vi "test.vi"() -> ()   [LabVIEW 2016]
uses:
  common_labview_tcpdevice/ts_labview_tcp/tcpTypedefs/TCPSettings.ctl
  IDome/domeTypedefs/azimuth.ctl
  domeCommunicator/ComTypedefs/shortStatus.ctl
  domeCommunicator/ComTypedefs/openingStates.ctl
  IDome/domeTypedefs/openingPercentage.ctl
  domeCommunicator/ComTypedefs/sensorCode.ctl
  domeCommunicator/ComTypedefs/azimimuthPositionStatus.ctl
  IDome/domeTypedefs/direction.ctl
  IDome/domeTypedefs/domeState.ctl
  IDome/domeTypedefs/motionDirection.ctl
  IDome/domeTypedefs/openingMotion.ctl
  domeCommunicator/ComTypedefs/engineeringStatus.ctl
  domeCommunicator/ATDomeCommunicator.lvclass
  domeController/DomeController.lvclass
  domeCommunicator/ComTypedefs/queries.ctl
  domeCommunicator/ComTypedefs/commands.ctl
panel:
  out "Timeout":errorcluster
  in  "TCP Settings":T1={"IP"="192.168.222.77", "port_low"=17310, "port_up"=17310, "connection_timeout "=1500, "reading_timeout"=1500, "writing_timeout"=1500}
  out "Connected":bool
  in  "disconnect":bool
  in  "connect":bool
  in  "azimuth":T2 min=0.0 max=360.0
  in  "SynchronizedClose":bool
  in  "MoveToAzimuth":bool
  in  "Synchronized Open":bool
  in  "StopAllMotion":bool
  in  "stop":bool
  in  "GetCurrentConfiguration":bool
  in  "SaveCurrentConfiguration":bool
  in  "reverseMotionDelay":dbl
  in  "ReverseMotionDelay":bool
  in  "watchDogTimer":u32
  in  "WatchdogTimer":bool
  in  "enconderCountPer360":dbl
  in  "EncoderCountPer360Deg":bool
  in  "coast":dbl
  in  "Coast":bool
  in  "highSpeedThreshold":dbl
  in  "HighSpeedThreshold":bool
  in  "homePosition":T2 min=0.0 max=360.0
  in  "SetHomePosition":bool
  in  "tolerance":dbl
  in  "Tolerance":bool
  in  "RotateToHomePosition":bool
  in  "CloudSensorOFF":bool
  in  "CloudSensorON":bool
  in  "RainSensorOFF":bool
  in  "CloseMainDoor":bool
  in  "RainSensorON":bool
  in  "AutoShutdownOFF":bool
  in  "AutoShutdownON":bool
  in  "CloseDropoutDoor":bool
  in  "OpenDropoutDoor":bool
  in  "OpenMainDoor":bool
  in  "Status":enum32{"Status", "Detailed Status"}(tab)
  out "shortStatus":T3 {"azimuthAngle" min=0.0 max=360.0; "dropoutDoorOpeningPercentage" min=0.0 max=100.0; "mainDoorOpeningPercentage" min=0.0 max=100.0}
  out "engineeringStatus":T12
  out "Disconnect":errorcluster
  # "Settings"
  # "Main Controls"
  # "degrees"
  # "Advanced Controls"
  # "degrees"
  # "degrees"
  # "degrees"
  # "degrees"
  # "counts"
  # "seconds"
  # "seconds"
  # "Save file to cRio"
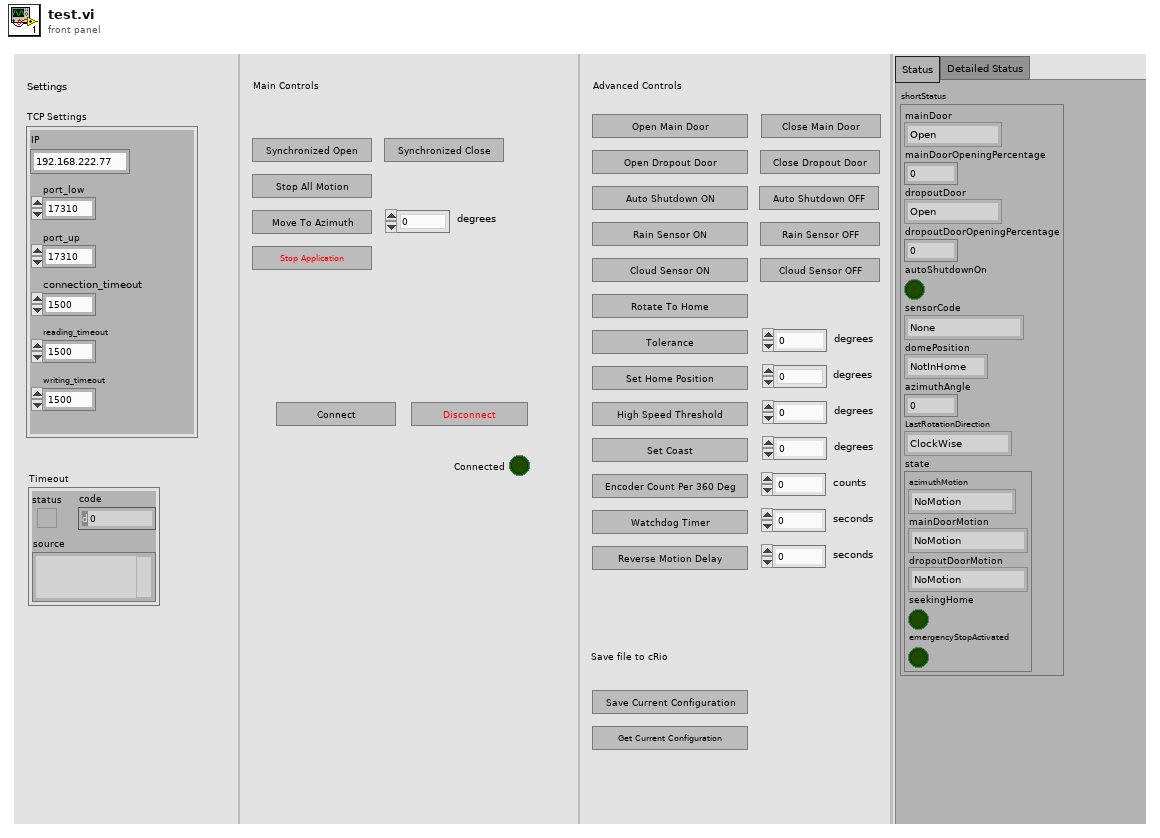
[diagram p1: front panel]
types:
  T1 = typedef "TCPSettings.ctl" = cluster{"IP":string, "port_low":u16, "port_up":u16, "connection_timeout ":i32, "reading_timeout":i32, "writing_timeout":i32}
  T2 = typedef "azimuth.ctl" = dbl
  T3 = typedef "shortStatus.ctl" = cluster{"mainDoor":T4, "mainDoorOpeningPercentage":T5, "dropoutDoor":T4, "dropoutDoorOpeningPercentage":T5, "autoShutdownOn":bool, "sensorCode":T6, "domePosition":T7, "azimuthAngle":T2, "LastRotationDirection":T8, "state":T9}
  T4 = typedef "openingStates.ctl" = enum16{"Open", "Shut", "Ajar"}
  T5 = typedef "openingPercentage.ctl" = dbl
  T6 = typedef "sensorCode.ctl" = enum16{"None", "RainSnowSensorTriggered", "CloudSensorTriggered", "BothSensorsTriggered"}
  T7 = typedef "azimimuthPositionStatus.ctl" = enum16{"NotInHome", "Home"}
  T8 = typedef "direction.ctl" = enum16{"ClockWise", "CounterClockWise"}
  T9 = typedef "domeState.ctl" = cluster{"azimuthMotion":T10, "mainDoorMotion":T11, "dropoutDoorMotion ":T11, "seekingHome":bool, "emergencyStopActivated":bool}
  T10 = typedef "motionDirection.ctl" = enum16{"NoMotion", "MovingClockWise", "MovingCounterClockWise"}
  T11 = typedef "openingMotion.ctl" = enum16{"NoMotion", "Opening", "Closing"}
  T12 = typedef "engineeringStatus.ctl" = cluster{"SCBRatioLinkOK":bool, "homeAzimuth":dbl, "highSpeed":dbl, "coast":dbl, "tolerance":dbl, "enconderCountPer360":u32, "encoderCount":u32, "lastAzimuthGoTo":dbl, "rainSnowSensoEnabled":bool, "cloudSensorEnabled":bool, "watchdogResetTime":dbl, "dropoutTimer":dbl, "reverseDelay":dbl, "mainDoorEncoderClosed":u32, "mainDoorEncoderOpened":u32, "dropoutEncoderClosed":u32, "dropoutEncoderOpened":u32}
  T13 = typedef "queries.ctl" = enum16{"ShortStatus", "FullEngineeringStatus", "RecallLastSavedConfiguration"}
  T14 = typedef "commands.ctl" = enum16{"StopAllMotion", "CloseMainDoor", "OpenMainDoor", "CloseDropoutDoor", "OpenDropoutDoor", "SynchronizedOpen", "SynchronizedClose", "AutoShutDownOn", "AutoShutDownOff", "RainOn", "RainOff", "CloudSensorOn", "CloudSensorOff", "RotateToHomePosition", "MoveToAzimuth", "SetTolerance", "DefineHomePosition", "HighSpeedThreshold", "SetCoast", "SetEncoderCountFor360", "SetWatchDogTimer", "SetReverseDirectionMotionDelay", "SaveCurrentConfiguration"}
  T15 = typedef "fullEngineeringStatus.ctl" = cluster{"shortStatus":T3, "engineeringStatus":T12}
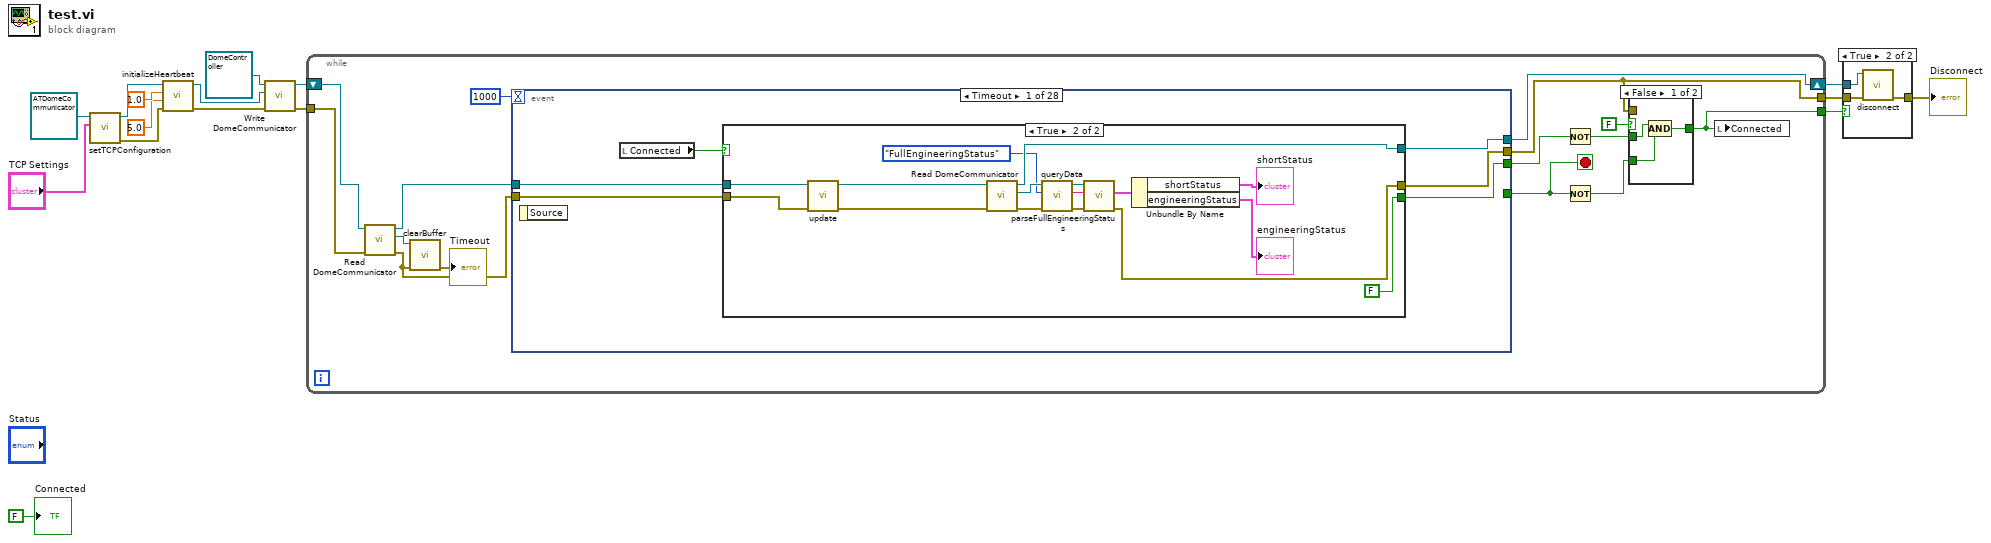
[diagram p0: block diagram]
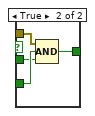
[diagram p3: hidden frame]
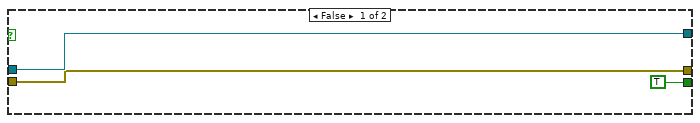
[diagram p4: hidden frame]
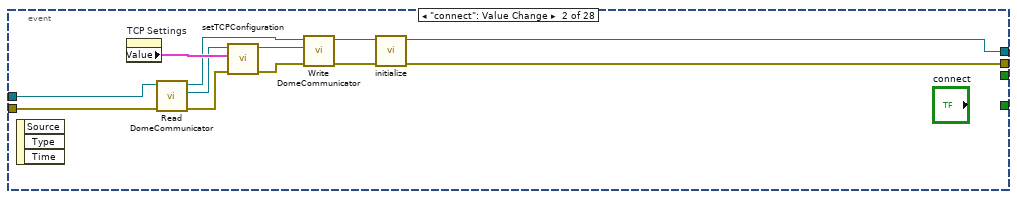
[diagram p5: hidden frame]
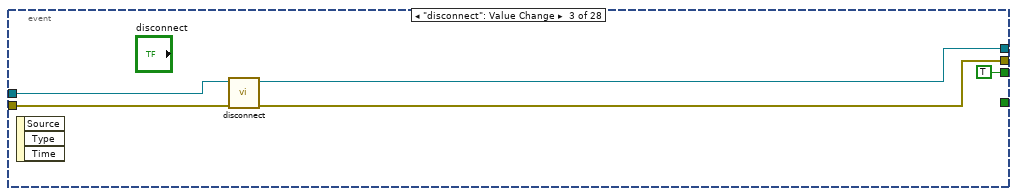
[diagram p6: hidden frame]
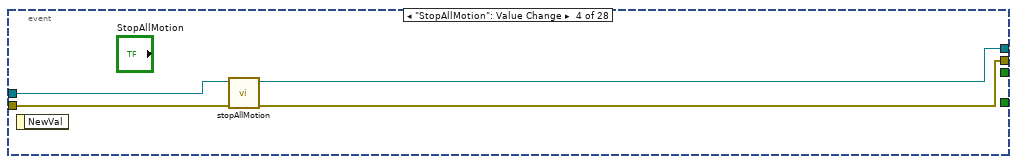
[diagram p7: hidden frame]
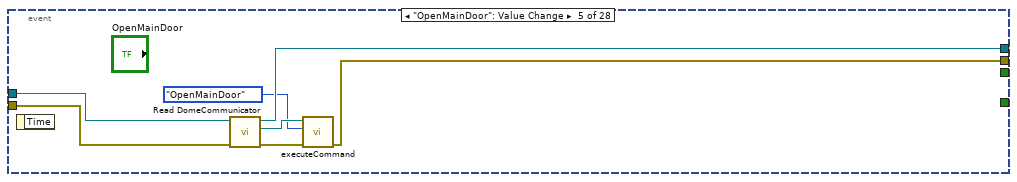
[diagram p8: hidden frame]
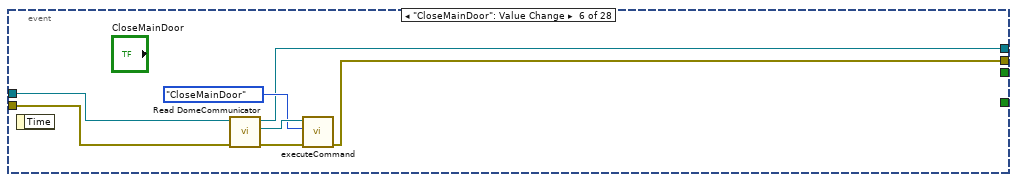
[diagram p9: hidden frame]
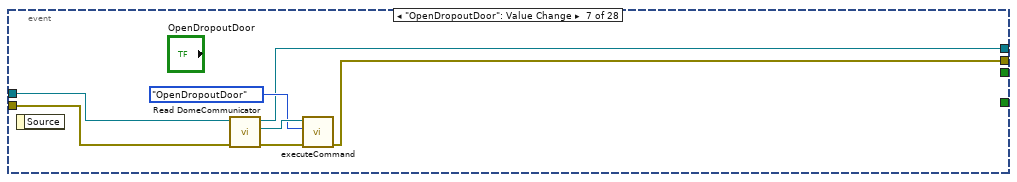
[diagram p10: hidden frame]
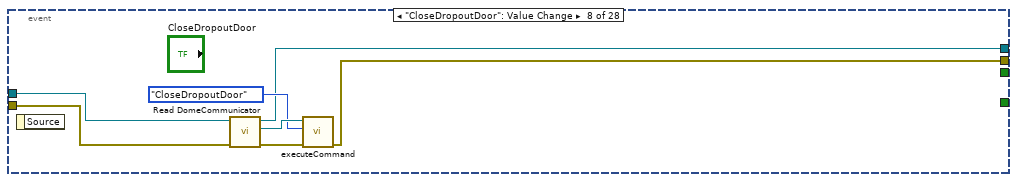
[diagram p11: hidden frame]
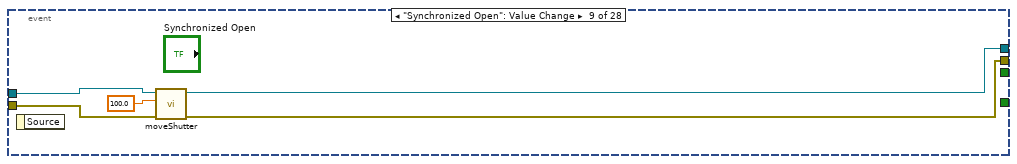
[diagram p12: hidden frame]
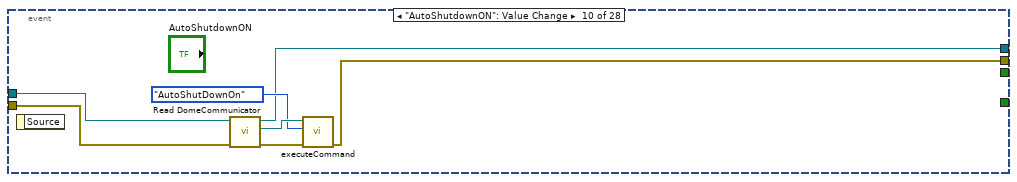
[diagram p13: hidden frame]
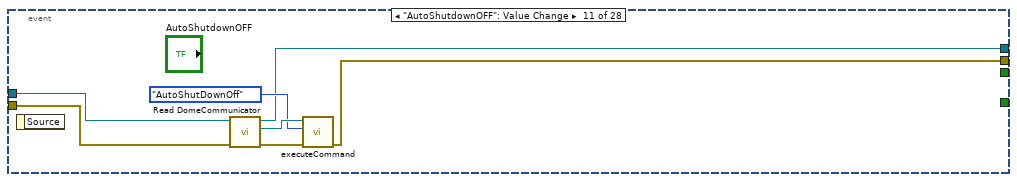
[diagram p14: hidden frame]
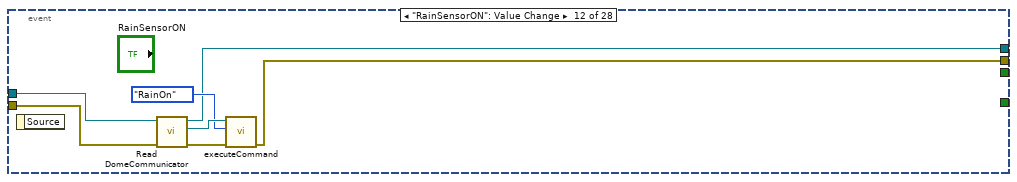
[diagram p15: hidden frame]
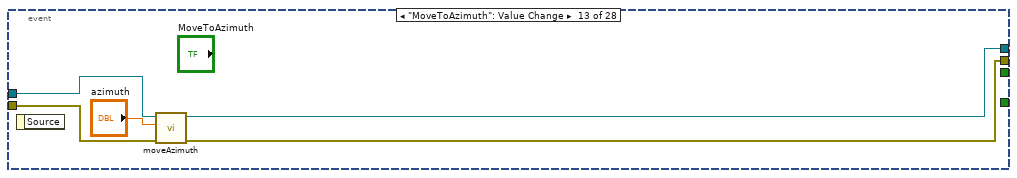
[diagram p16: hidden frame]
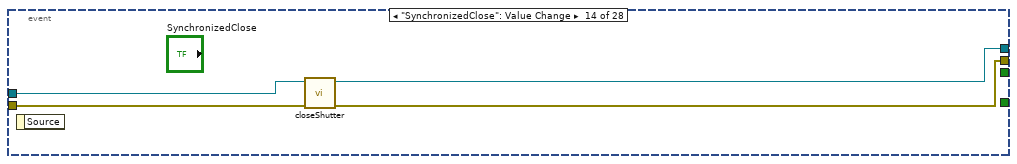
[diagram p17: hidden frame]
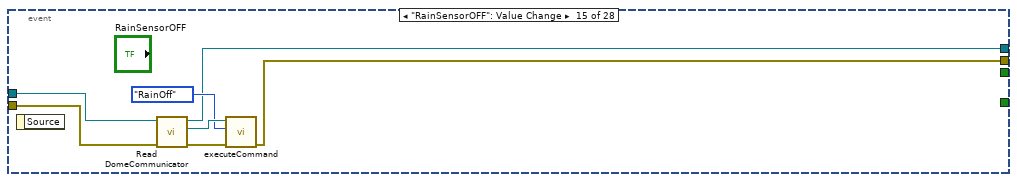
[diagram p18: hidden frame]
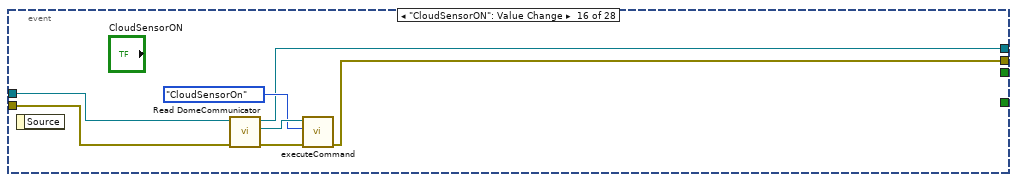
[diagram p19: hidden frame]
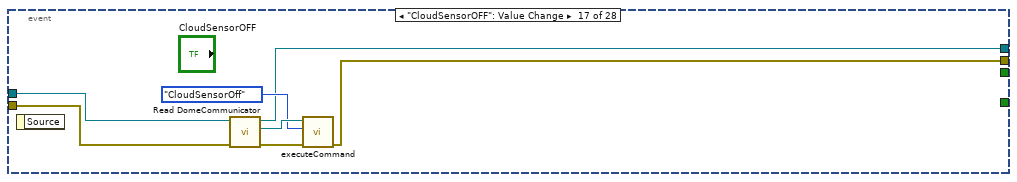
[diagram p20: hidden frame]
diagram:
  n1 = call-dynamic "setTCPConfiguration.vi"("Settings"="TCP Settings", "tcpDevice in"=refnum<class "ATDomeCommunicator.lvclass"> refnum ("domeCommunicator.lvclass")) -> ("error out"=w5:errorcluster, "tcpDevice out"=w6:refnum<class "ATDomeCommunicator.lvclass">)  [unwired: 8 in]
  n2 = call-dynamic "initializeHeartbeat.vi"("error in (no error)"=w5, "timeout"=5.0, "period"=1.0, "tcpDevice in"=w6) -> ("error out"=w10:errorcluster, "tcpDevice out"=w9:refnum<class "ATDomeCommunicator.lvclass">)  [unwired: 6 in]
  n3 = call-dynamic "Write DomeCommunicator.vi"("error in (no error)"=w10, "DomeCommunicator.lvclass"=w9, "DomeController in"=refnum<class "DomeController.lvclass"> refnum) -> ("error out"=w3:errorcluster, "DomeController out"=w4:refnum<class "DomeController.lvclass">)  [unwired: 7 in]
  n4 = while {
    tunnel: w3 -> [w20]
    tunnel: [w24] -> w12
    shift-right: [w30] -> w7
    shift-left: w4 -> [w22]
    tunnel: [w25] -> w2
    stop <- w29 stop-if-true
    n5 = call-dynamic "Read DomeCommunicator.vi"("error in (no error)"=w20, "DomeController in"=w22) -> ("error out"=w18:errorcluster, "DomeCommunicator.lvclass"=w19:refnum<class "ATDomeCommunicator.lvclass">, "DomeController out"=w21:refnum<class "DomeController.lvclass">)  [unwired: 7 in]
    n6 = call "clearBuffer.vi"("error in (no error)"=w18, "DomeCommunicator in"=w19) -> ("error out"=→"Timeout":errorcluster)  [unwired: 6 in, 3 out]
    n7 = event shown="[0] Timeout" {
      selector: _ -> [_ _ _ _ _ _ _ _ _ _ _ _ _ _ _ _ _ _ _ _ _ _ _ _ _ _ _ _]
      dyn-events: _ -> [_ _ _ _ _ _ _ _ _ _ _ _ _ _ _ _ _ _ _ _ _ _ _ _ _ _ _ _]
      timeout: 1000 -> [_ _ _ _ _ _ _ _ _ _ _ _ _ _ _ _ _ _ _ _ _ _ _ _ _ _ _ _]
      tunnel: w18 -> [w43 w67 w79 w83 w90 w95 w101 w108 w116 w120 w127 w134 w141 w146 w150 w157 w164 w171 w180 w187 w195 w203 w211 w219 w227 w234 w246 w247]
      tunnel: w21 -> [w44 w68 w80 w84 w91 w94 w102 w109 w117 w121 w128 w135 w143 w147 w151 w158 w165 w172 w179 w188 w196 w204 w212 w220 w228 w235 w245 w248]
      tunnel: [w42 w74 w77 w81 w86 w93 w99 w106 w114 w118 w125 w132 w142 w144 w148 w155 w162 w169 w178 w185 w193 w201 w209 w217 w225 w232 w244 w248] -> w30
      tunnel: [w41 w75 w78 w82 w87 w92 w100 w107 w115 w119 w126 w133 w139 w145 w149 w156 w163 w170 w177 w186 w194 w202 w210 w218 w226 w233 w240 w247] -> w24
      tunnel: [_ _ _ _ _ _ _ _ _ _ _ _ _ _ _ _ _ _ _ _ _ _ _ _ _ _ _ "stop"] -> w29
      tunnel: [w39 _ TRUE ("stop") _ _ _ _ _ _ _ _ _ _ _ _ _ _ _ _ _ _ _ _ _ _ _ _ _] -> w27
      event Timeout {
        n8 = event-data() -> ()  [unwired: 1 in, 1 out]
        n9 = local read "Connected"() -> (w40:bool)
        n10 = case shown="True" w40 {
          tunnel: w44 -> [w47 w63]
          tunnel: w43 -> [w46 w62]
          tunnel: [w47 w59] -> w42
          tunnel: [w46 w54] -> w41
          tunnel: [TRUE ("stop") FALSE ("stop")] -> w39
          frame False {
          }
          frame True {
            n11 = call-dynamic "update.vi"("error in (no error)"=w62, "DomeController in"=w63) -> ("error out"=w60:errorcluster, "DomeController out"=w61:refnum<class "DomeController.lvclass">)  [unwired: 6 in, 2 out]
            n12 = call-dynamic "Read DomeCommunicator.vi"("error in (no error)"=w60, "DomeController in"=w61) -> ("error out"=w57:errorcluster, "DomeCommunicator.lvclass"=w58:refnum<class "ATDomeCommunicator.lvclass">, "DomeController out"=w59:refnum<class "DomeController.lvclass">)  [unwired: 7 in]
            n13 = call "queryData.vi"("error in (no error)"=w57, "queries"=queries."FullEngineeringStatus", "DomeCommunicator in"=w58) -> ("error out"=w55:errorcluster, "response"=w52:string, "DomeCommunicator out"=w53:refnum<class "ATDomeCommunicator.lvclass">)  [unwired: 5 in, 1 out]
            n14 = call "parseFullEngineeringStatus.vi"("error in (no error)"=w55, "engineeringStatusString"=w52, "DomeCommunicator in"=w53) -> ("error out"=w54:errorcluster, "fullEngineeringStatus"=w51:T15)  [unwired: 6 in, 1 out]
            n15 = Unbundle By Name(w51) -> ("shortStatus"=→"shortStatus":T3, "engineeringStatus"=→"engineeringStatus":T12)
          }
        }
      }
      event "connect": Value Change {
        n16 = event-data() -> ()  [unwired: 1 in, 3 out]
        n17 = property on="TCP Settings" class="Clust (strict)"() -> ("Value"=w69:T1)  [unwired: 2 in, 2 out]
        n18 = call-dynamic "Read DomeCommunicator.vi"("error in (no error)"=w67, "DomeController in"=w68) -> ("error out"=w64:errorcluster, "DomeCommunicator.lvclass"=w66:refnum<class "ATDomeCommunicator.lvclass">, "DomeController out"=w65:refnum<class "DomeController.lvclass">)  [unwired: 7 in]
        n19 = call-dynamic "setTCPConfiguration.vi"("error in (no error)"=w64, "Settings"=w69, "tcpDevice in"=w66) -> ("error out"=w73:errorcluster, "tcpDevice out"=w70:refnum<class "ATDomeCommunicator.lvclass">)  [unwired: 7 in]
        n20 = call-dynamic "Write DomeCommunicator.vi"("error in (no error)"=w73, "DomeCommunicator.lvclass"=w70, "DomeController in"=w65) -> ("error out"=w72:errorcluster, "DomeController out"=w71:refnum<class "DomeController.lvclass">)  [unwired: 7 in]
        n21 = call-dynamic "initialize.vi"("error in (no error)"=w72, "DomeController in"=w71) -> ("error out"=w75:errorcluster, "DomeController out"=w74:refnum<class "DomeController.lvclass">)  [unwired: 8 in]
      }
      event "disconnect": Value Change {
        n22 = event-data() -> ()  [unwired: 1 in, 3 out]
        n23 = call-dynamic "disconnect.vi"("error in (no error)"=w79, "DomeController in"=w80) -> ("error out"=w78:errorcluster, "DomeController out"=w77:refnum<class "DomeController.lvclass">)  [unwired: 8 in]
      }
      event "StopAllMotion": Value Change {
        n24 = event-data() -> ()  [unwired: 1 in, 1 out]
        n25 = call-dynamic "stopAllMotion.vi"("error in (no error)"=w83, "DomeController in"=w84) -> ("error out"=w82:errorcluster, "DomeController out"=w81:refnum<class "DomeController.lvclass">)  [unwired: 8 in]
      }
      event "OpenMainDoor": Value Change {
        n26 = event-data() -> ()  [unwired: 1 in, 1 out]
        n27 = call-dynamic "Read DomeCommunicator.vi"("error in (no error)"=w90, "DomeController in"=w91) -> ("error out"=w88:errorcluster, "DomeCommunicator.lvclass"=w89:refnum<class "ATDomeCommunicator.lvclass">, "DomeController out"=w86:refnum<class "DomeController.lvclass">)  [unwired: 7 in]
        n28 = call "executeCommand.vi"("error in (no error)"=w88, "Command"=commands."OpenMainDoor", "DomeCommunicator in"=w89) -> ("error out"=w87:errorcluster)  [unwired: 7 in, 1 out]
      }
      event "CloseMainDoor": Value Change {
        n29 = event-data() -> ()  [unwired: 1 in, 1 out]
        n30 = call-dynamic "Read DomeCommunicator.vi"("error in (no error)"=w95, "DomeController in"=w94) -> ("error out"=w97:errorcluster, "DomeCommunicator.lvclass"=w98:refnum<class "ATDomeCommunicator.lvclass">, "DomeController out"=w93:refnum<class "DomeController.lvclass">)  [unwired: 7 in]
        n31 = call "executeCommand.vi"("error in (no error)"=w97, "Command"=commands."CloseMainDoor", "DomeCommunicator in"=w98) -> ("error out"=w92:errorcluster)  [unwired: 7 in, 1 out]
      }
      event "OpenDropoutDoor": Value Change {
        n32 = event-data() -> ()  [unwired: 1 in, 1 out]
        n33 = call-dynamic "Read DomeCommunicator.vi"("error in (no error)"=w101, "DomeController in"=w102) -> ("error out"=w104:errorcluster, "DomeCommunicator.lvclass"=w105:refnum<class "ATDomeCommunicator.lvclass">, "DomeController out"=w99:refnum<class "DomeController.lvclass">)  [unwired: 7 in]
        n34 = call "executeCommand.vi"("error in (no error)"=w104, "Command"=commands."OpenDropoutDoor", "DomeCommunicator in"=w105) -> ("error out"=w100:errorcluster)  [unwired: 7 in, 1 out]
      }
      event "CloseDropoutDoor": Value Change {
        n35 = event-data() -> ()  [unwired: 1 in, 1 out]
        n36 = call-dynamic "Read DomeCommunicator.vi"("error in (no error)"=w108, "DomeController in"=w109) -> ("error out"=w111:errorcluster, "DomeCommunicator.lvclass"=w112:refnum<class "ATDomeCommunicator.lvclass">, "DomeController out"=w106:refnum<class "DomeController.lvclass">)  [unwired: 7 in]
        n37 = call "executeCommand.vi"("error in (no error)"=w111, "Command"=commands."CloseDropoutDoor", "DomeCommunicator in"=w112) -> ("error out"=w107:errorcluster)  [unwired: 7 in, 1 out]
      }
      event "Synchronized Open": Value Change {
        n38 = event-data() -> ()  [unwired: 1 in, 1 out]
        n39 = call-dynamic "moveShutter.vi"("error in (no error)"=w116, "openingPercentage"=T5 100.0, "DomeController in"=w117) -> ("error out"=w115:errorcluster, "DomeController out"=w114:refnum<class "DomeController.lvclass">)  [unwired: 7 in]
      }
      event "AutoShutdownON": Value Change {
        n40 = event-data() -> ()  [unwired: 1 in, 1 out]
        n41 = call-dynamic "Read DomeCommunicator.vi"("error in (no error)"=w120, "DomeController in"=w121) -> ("error out"=w123:errorcluster, "DomeCommunicator.lvclass"=w124:refnum<class "ATDomeCommunicator.lvclass">, "DomeController out"=w118:refnum<class "DomeController.lvclass">)  [unwired: 7 in]
        n42 = call "executeCommand.vi"("error in (no error)"=w123, "Command"=commands."AutoShutDownOn", "DomeCommunicator in"=w124) -> ("error out"=w119:errorcluster)  [unwired: 7 in, 1 out]
      }
      event "AutoShutdownOFF": Value Change {
        n43 = event-data() -> ()  [unwired: 1 in, 1 out]
        n44 = call-dynamic "Read DomeCommunicator.vi"("error in (no error)"=w127, "DomeController in"=w128) -> ("error out"=w130:errorcluster, "DomeCommunicator.lvclass"=w131:refnum<class "ATDomeCommunicator.lvclass">, "DomeController out"=w125:refnum<class "DomeController.lvclass">)  [unwired: 7 in]
        n45 = call "executeCommand.vi"("error in (no error)"=w130, "Command"=commands."AutoShutDownOff", "DomeCommunicator in"=w131) -> ("error out"=w126:errorcluster)  [unwired: 7 in, 1 out]
      }
      event "RainSensorON": Value Change {
        n46 = event-data() -> ()  [unwired: 1 in, 1 out]
        n47 = call-dynamic "Read DomeCommunicator.vi"("error in (no error)"=w134, "DomeController in"=w135) -> ("error out"=w137:errorcluster, "DomeCommunicator.lvclass"=w138:refnum<class "ATDomeCommunicator.lvclass">, "DomeController out"=w132:refnum<class "DomeController.lvclass">)  [unwired: 7 in]
        n48 = call "executeCommand.vi"("error in (no error)"=w137, "Command"=commands."RainOn", "DomeCommunicator in"=w138) -> ("error out"=w133:errorcluster)  [unwired: 7 in, 1 out]
      }
      event "MoveToAzimuth": Value Change {
        n49 = event-data() -> ()  [unwired: 1 in, 1 out]
        n50 = call-dynamic "moveAzimuth.vi"("error in (no error)"=w141, "azimuth"="azimuth", "DomeController in"=w143) -> ("error out"=w139:errorcluster, "DomeController out"=w142:refnum<class "DomeController.lvclass">)  [unwired: 7 in]
      }
      event "SynchronizedClose": Value Change {
        n51 = event-data() -> ()  [unwired: 1 in, 1 out]
        n52 = call-dynamic "closeShutter.vi"("error in (no error)"=w146, "DomeController in"=w147) -> ("error out"=w145:errorcluster, "DomeController out"=w144:refnum<class "DomeController.lvclass">)  [unwired: 8 in]
      }
      event "RainSensorOFF": Value Change {
        n53 = event-data() -> ()  [unwired: 1 in, 1 out]
        n54 = call-dynamic "Read DomeCommunicator.vi"("error in (no error)"=w150, "DomeController in"=w151) -> ("error out"=w153:errorcluster, "DomeCommunicator.lvclass"=w154:refnum<class "ATDomeCommunicator.lvclass">, "DomeController out"=w148:refnum<class "DomeController.lvclass">)  [unwired: 7 in]
        n55 = call "executeCommand.vi"("error in (no error)"=w153, "Command"=commands."RainOff", "DomeCommunicator in"=w154) -> ("error out"=w149:errorcluster)  [unwired: 7 in, 1 out]
      }
      event "CloudSensorON": Value Change {
        n56 = event-data() -> ()  [unwired: 1 in, 1 out]
        n57 = call-dynamic "Read DomeCommunicator.vi"("error in (no error)"=w157, "DomeController in"=w158) -> ("error out"=w160:errorcluster, "DomeCommunicator.lvclass"=w161:refnum<class "ATDomeCommunicator.lvclass">, "DomeController out"=w155:refnum<class "DomeController.lvclass">)  [unwired: 7 in]
        n58 = call "executeCommand.vi"("error in (no error)"=w160, "Command"=commands."CloudSensorOn", "DomeCommunicator in"=w161) -> ("error out"=w156:errorcluster)  [unwired: 7 in, 1 out]
      }
      event "CloudSensorOFF": Value Change {
        n59 = event-data() -> ()  [unwired: 1 in, 1 out]
        n60 = call-dynamic "Read DomeCommunicator.vi"("error in (no error)"=w164, "DomeController in"=w165) -> ("error out"=w167:errorcluster, "DomeCommunicator.lvclass"=w168:refnum<class "ATDomeCommunicator.lvclass">, "DomeController out"=w162:refnum<class "DomeController.lvclass">)  [unwired: 7 in]
        n61 = call "executeCommand.vi"("error in (no error)"=w167, "Command"=commands."CloudSensorOff", "DomeCommunicator in"=w168) -> ("error out"=w163:errorcluster)  [unwired: 7 in, 1 out]
      }
      event "RotateToHomePosition": Value Change {
        n62 = event-data() -> ()  [unwired: 1 in, 1 out]
        n63 = call-dynamic "Read DomeCommunicator.vi"("error in (no error)"=w171, "DomeController in"=w172) -> ("error out"=w174:errorcluster, "DomeCommunicator.lvclass"=w175:refnum<class "ATDomeCommunicator.lvclass">, "DomeController out"=w169:refnum<class "DomeController.lvclass">)  [unwired: 7 in]
        n64 = call "executeCommand.vi"("error in (no error)"=w174, "Command"=commands."RotateToHomePosition", "DomeCommunicator in"=w175) -> ("error out"=w170:errorcluster)  [unwired: 7 in, 1 out]
      }
      event "Tolerance": Value Change {
        n65 = event-data() -> ()  [unwired: 1 in, 1 out]
        n66 = call-dynamic "Read DomeCommunicator.vi"("error in (no error)"=w180, "DomeController in"=w179) -> ("error out"=w182:errorcluster, "DomeCommunicator.lvclass"=w183:refnum<class "ATDomeCommunicator.lvclass">, "DomeController out"=w178:refnum<class "DomeController.lvclass">)  [unwired: 7 in]
        n67 = call "executeCommand.vi"("error in (no error)"=w182, "Variant"="tolerance", "Command"=commands."SetTolerance", "DomeCommunicator in"=w183) -> ("error out"=w177:errorcluster)  [unwired: 6 in, 1 out]
      }
      event "SetHomePosition": Value Change {
        n68 = event-data() -> ()  [unwired: 1 in, 1 out]
        n69 = call-dynamic "Read DomeCommunicator.vi"("error in (no error)"=w187, "DomeController in"=w188) -> ("error out"=w190:errorcluster, "DomeCommunicator.lvclass"=w191:refnum<class "ATDomeCommunicator.lvclass">, "DomeController out"=w185:refnum<class "DomeController.lvclass">)  [unwired: 7 in]
        n70 = call "executeCommand.vi"("error in (no error)"=w190, "Variant"="homePosition", "Command"=commands."DefineHomePosition", "DomeCommunicator in"=w191) -> ("error out"=w186:errorcluster)  [unwired: 6 in, 1 out]
      }
      event "HighSpeedThreshold": Value Change {
        n71 = event-data() -> ()  [unwired: 1 in, 1 out]
        n72 = call-dynamic "Read DomeCommunicator.vi"("error in (no error)"=w195, "DomeController in"=w196) -> ("error out"=w198:errorcluster, "DomeCommunicator.lvclass"=w199:refnum<class "ATDomeCommunicator.lvclass">, "DomeController out"=w193:refnum<class "DomeController.lvclass">)  [unwired: 7 in]
        n73 = call "executeCommand.vi"("error in (no error)"=w198, "Variant"="highSpeedThreshold", "Command"=commands."HighSpeedThreshold", "DomeCommunicator in"=w199) -> ("error out"=w194:errorcluster)  [unwired: 6 in, 1 out]
      }
      event "Coast": Value Change {
        n74 = event-data() -> ()  [unwired: 1 in, 1 out]
        n75 = call-dynamic "Read DomeCommunicator.vi"("error in (no error)"=w203, "DomeController in"=w204) -> ("error out"=w206:errorcluster, "DomeCommunicator.lvclass"=w207:refnum<class "ATDomeCommunicator.lvclass">, "DomeController out"=w201:refnum<class "DomeController.lvclass">)  [unwired: 7 in]
        n76 = call "executeCommand.vi"("error in (no error)"=w206, "Variant"="coast", "Command"=commands."SetCoast", "DomeCommunicator in"=w207) -> ("error out"=w202:errorcluster)  [unwired: 6 in, 1 out]
      }
      event "EncoderCountPer360Deg": Value Change {
        n77 = event-data() -> ()  [unwired: 1 in, 1 out]
        n78 = call-dynamic "Read DomeCommunicator.vi"("error in (no error)"=w211, "DomeController in"=w212) -> ("error out"=w214:errorcluster, "DomeCommunicator.lvclass"=w215:refnum<class "ATDomeCommunicator.lvclass">, "DomeController out"=w209:refnum<class "DomeController.lvclass">)  [unwired: 7 in]
        n79 = call "executeCommand.vi"("error in (no error)"=w214, "Variant"="enconderCountPer360", "Command"=commands."SetEncoderCountFor360", "DomeCommunicator in"=w215) -> ("error out"=w210:errorcluster)  [unwired: 6 in, 1 out]
      }
      event "WatchdogTimer": Value Change {
        n80 = event-data() -> ()  [unwired: 1 in, 1 out]
        n81 = call-dynamic "Read DomeCommunicator.vi"("error in (no error)"=w219, "DomeController in"=w220) -> ("error out"=w222:errorcluster, "DomeCommunicator.lvclass"=w223:refnum<class "ATDomeCommunicator.lvclass">, "DomeController out"=w217:refnum<class "DomeController.lvclass">)  [unwired: 7 in]
        n82 = call "executeCommand.vi"("error in (no error)"=w222, "Variant"="watchDogTimer", "Command"=commands."SetWatchDogTimer", "DomeCommunicator in"=w223) -> ("error out"=w218:errorcluster)  [unwired: 6 in, 1 out]
      }
      event "ReverseMotionDelay": Value Change {
        n83 = event-data() -> ()  [unwired: 1 in, 1 out]
        n84 = call-dynamic "Read DomeCommunicator.vi"("error in (no error)"=w227, "DomeController in"=w228) -> ("error out"=w230:errorcluster, "DomeCommunicator.lvclass"=w231:refnum<class "ATDomeCommunicator.lvclass">, "DomeController out"=w225:refnum<class "DomeController.lvclass">)  [unwired: 7 in]
        n85 = call "executeCommand.vi"("error in (no error)"=w230, "Variant"="reverseMotionDelay", "Command"=commands."SetReverseDirectionMotionDelay", "DomeCommunicator in"=w231) -> ("error out"=w226:errorcluster)  [unwired: 6 in, 1 out]
      }
      event "SaveCurrentConfiguration": Value Change {
        n86 = event-data() -> ()  [unwired: 1 in, 1 out]
        n87 = call-dynamic "Read DomeCommunicator.vi"("error in (no error)"=w234, "DomeController in"=w235) -> ("error out"=w237:errorcluster, "DomeCommunicator.lvclass"=w238:refnum<class "ATDomeCommunicator.lvclass">, "DomeController out"=w232:refnum<class "DomeController.lvclass">)  [unwired: 7 in]
        n88 = call "executeCommand.vi"("error in (no error)"=w237, "Command"=commands."SaveCurrentConfiguration", "DomeCommunicator in"=w238) -> ("error out"=w233:errorcluster)  [unwired: 7 in, 1 out]
      }
      event "GetCurrentConfiguration": Value Change {
        n89 = event-data() -> ()  [unwired: 1 in, 1 out]
        n90 = call-dynamic "Read DomeCommunicator.vi"("error in (no error)"=w246, "DomeController in"=w245) -> ("error out"=w242:errorcluster, "DomeCommunicator.lvclass"=w243:refnum<class "ATDomeCommunicator.lvclass">, "DomeController out"=w244:refnum<class "DomeController.lvclass">)  [unwired: 7 in]
        n91 = call "queryData.vi"("error in (no error)"=w242, "queries"=queries."RecallLastSavedConfiguration", "DomeCommunicator in"=w243) -> ("error out"=w240:errorcluster, "response"=w239:string)  [unwired: 5 in, 2 out]
        n92 = call "Display Message to User"("Message"=w239) -> ()  [unwired: 9 in, 2 out]
      }
      event "stop": Value Change {
        n93 = event-data() -> ()  [unwired: 1 in, 1 out]
      }
    }
    n94 = Not(x=w27) -> (.not. x?=w26:bool)
    n95 = Not(x=w29) -> (.not. x?=w28:bool)
    n96 = case shown="False" FALSE {
      tunnel: w28 -> [w32 w38]
      tunnel: w26 -> [w33 w37]
      tunnel: [w34 w36] -> w25
      tunnel: w24 -> [_ w35]
      frame False {
        n97 = Compound Arithmetic op=AND(w33, w32) -> (w34:bool)
      }
      frame True {
        n98 = Compound Arithmetic op=AND(w35, w38, w37) -> (w36:bool)
      }
    }
    n99 = local write "Connected"(w25) -> ()
  }
  n100 = case shown="True" w2 {
    tunnel: w12 -> [w250 w253]
    tunnel: [w250 w252] -> w11
    tunnel: w7 -> [_ w251]
    frame False {
    }
    frame True {
      n101 = call-dynamic "disconnect.vi"("error in (no error)"=w253, "DomeController in"=w251) -> ("error out"=w252:errorcluster)  [unwired: 8 in, 1 out]
    }
  }
  "Disconnect" <- w11
  "Connected" <- FALSE ("Connected")
